vi "Ask_Font.vi"(11 "WaveformGraph in":refnum<vi>) -> ()   [LabVIEW 2022 SP3]
uses:
  <vilib>/Utility/miscctls.llb/LVFontTypeDef.ctl
panel:
  in  "Y Scale":T1
  in  "OK Button":bool
  in  "Format":T1
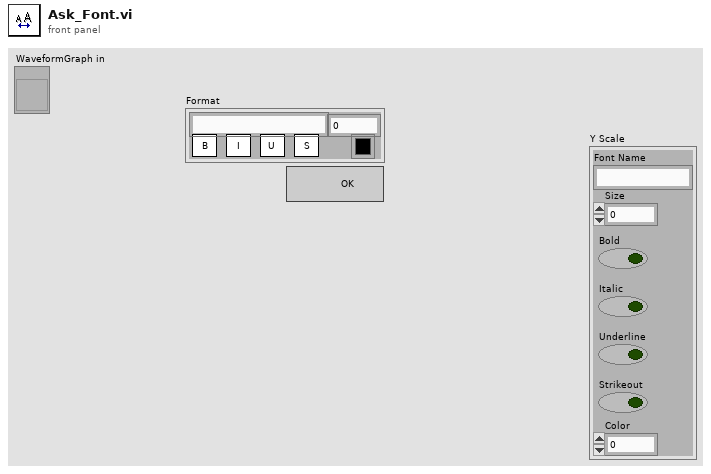
[diagram p1: front panel]
types:
  T1 = typedef "LVFontTypeDef.ctl" = cluster{"Font Name":string, "Size":u16, "Bold":bool, "Italic":bool, "Underline":bool, "Strikeout":bool, "Color":u32}
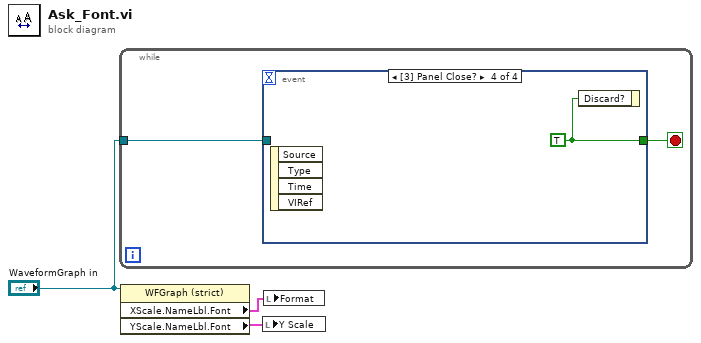
[diagram p0: block diagram]
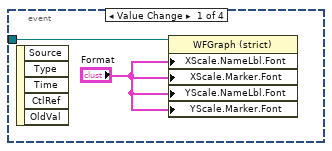
[diagram p2: hidden frame]
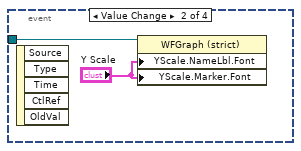
[diagram p3: hidden frame]
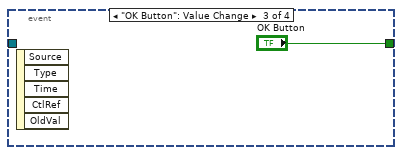
[diagram p4: hidden frame]
diagram:
  n1 = while {
    tunnel: "WaveformGraph in" -> [w5]
    stop <- w4 stop-if-true
    n2 = event shown="[3] Panel Close?" {
      selector: _ -> [_ _ _ _]
      dyn-events: _ -> [_ _ _ _]
      timeout: _ -> [_ _ _ _]
      tunnel: w5 -> [w7 w9 _ _]
      tunnel: [_ _ "OK Button" w11] -> w4
      event Value Change {
        n3 = event-data() -> ()  [unwired: 1 in, 5 out]
        n4 = property class="WFGraph (strict)"(reference=w7, "XScale.NameLbl.Font"="Format", "XScale.Marker.Font"="Format", "YScale.NameLbl.Font"="Format", "YScale.Marker.Font"="Format") -> ()  [unwired: 1 in, 2 out]
      }
      event Value Change {
        n5 = event-data() -> ()  [unwired: 1 in, 5 out]
        n6 = property class="WFGraph (strict)"(reference=w9, "YScale.NameLbl.Font"="Y Scale", "YScale.Marker.Font"="Y Scale") -> ()  [unwired: 1 in, 2 out]
      }
      event "OK Button": Value Change {
        n7 = event-data() -> ()  [unwired: 1 in, 5 out]
      }
      event Panel Close? {
        w11 = TRUE ("Discard?")
        n8 = event-data() -> ()  [unwired: 1 in, 4 out]
        n9 = event-data("Discard?"=w11) -> ()  [unwired: 1 in, 1 out]
      }
    }
  }
  n10 = property class="WFGraph (strict)"(reference="WaveformGraph in") -> ("XScale.NameLbl.Font"=w2:T1, "YScale.NameLbl.Font"=w1:T1)  [unwired: 1 in, 2 out]
  n11 = local write "Y Scale"(w1) -> ()
  n12 = local write "Format"(w2) -> ()
